vi "GlyphFactory_CleanUp.vi"(8 "error in (no error)":errorcluster) -> (0 "error out":errorcluster)   [LabVIEW 2012, in "GlyphFactory.lvclass"]
uses:
  GlyphFactory.lvclass
  Character_class/Character.lvclass
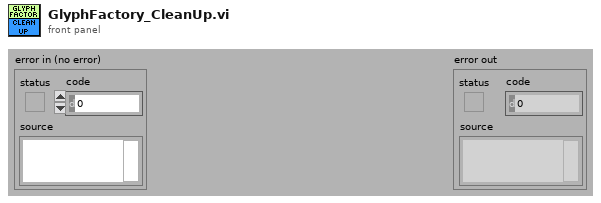
[diagram p1: front panel]
types:
  T1 = typedef "GlyphFactory.lvclass/ObjectAttributes.ctl" = cluster{"CharObjectTypes":cluster{"Char":string, "Text Color":u32, "Font":cluster{"Font Name:":string, "Size":i16, "Strikeout?":bool, "Italic?":bool, "Underline?":bool, "Outline?":bool, "Shadow?":bool, "Bold?":bool}}[], "CharObjects":refnum<class "Character.lvclass">[]}
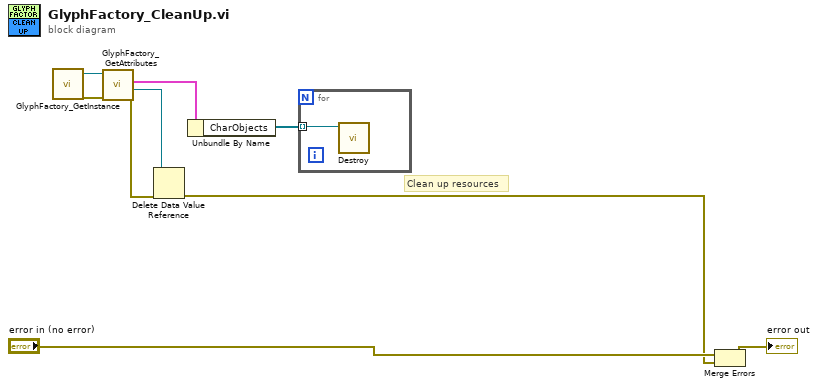
[diagram p0: block diagram]
diagram:
  # "Clean up resources"
  n1 = call "GlyphFactory_GetInstance.vi"() -> ("error out"=w7:errorcluster, "reference out"=w6:refnum<class "GlyphFactory.lvclass">)  [unwired: 8 in, 2 out]
  n2 = call "GlyphFactory_GetAttributes.vi"("error in (no error)"=w7, "reference in"=w6) -> ("error out"=w5:errorcluster, "DataRef"=w4:refnum<data-value>, "Data"=w8:T1)  [unwired: 6 in, 1 out]
  n3 = Delete Data Value Reference(data value reference=w4, error in=w5) -> (error out=w2:errorcluster)  [unwired: 1 out]
  n4 = Unbundle By Name(w8) -> ("CharObjects"=w1:refnum<class "Character.lvclass">[])
  n5 = for {
    tunnel: w1 -> [w10] mode=indexing
    n6 = call-dynamic "Destroy.vi"("reference in"=w10) -> ()  [unwired: 9 in, 2 out]
  }
  n7 = Merge Errors("error in (no error)", w2) -> (→"error out":errorcluster)
